vi "Set Channel Value and Get Buffer.vi"(8 "error in":errorcluster, 9 "Value":dbl, 10 "Channel":string, 11 "BufferWritesDBL in":refnum<class "BufferWrites1SamDBL.lvclass">) -> (0 "error out":errorcluster, 2 "Write Buffer":dbl[](array[numeric]), 3 "BufferWritesDBL out":refnum<class "BufferWrites1SamDBL.lvclass">)   [LabVIEW 2023, in "BufferWrites1SamDBL.lvclass"]
uses:
  BufferWrites1SamDBL.lvclass
  BufferWrites1SamDBL.lvclass/BufferWrites1SamDBL.ctl
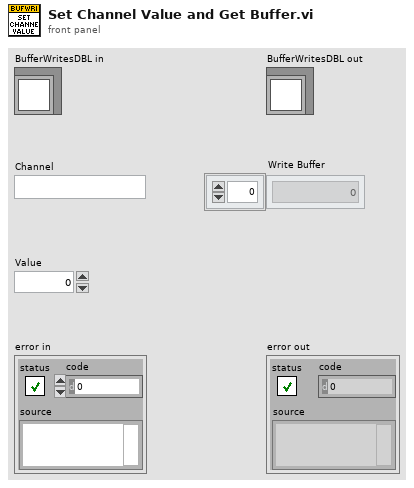
[diagram p1: front panel]
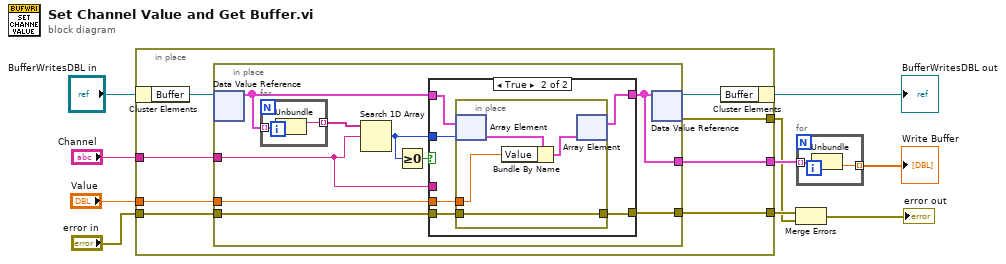
[diagram p0: block diagram]
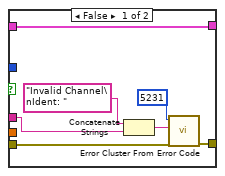
[diagram p2: hidden frame]
diagram:
  n1 = in-place {
    in-place-border: "Value" -> [w18]
    in-place-border: [w17] -> w1
    in-place-border: "Channel" -> [w16]
    in-place-border: [w13] -> w5
    in-place-border: "error in" -> [w12]
    in-place-border: [w11] -> w2
    n2 = in-place-cluster #1("BufferWritesDBL in") -> ("Buffer"=w15:refnum<data-value>)
    n3 = in-place {
      in-place-border: w18 -> [w27]
      in-place-border: w16 -> [w19]
      in-place-border: [w22] -> w13
      in-place-border: w12 -> [w21]
      in-place-border: [w20] -> w11
      n4 = in-place-dvr #2(w15) -> (w25:cluster{"Ident":string, "Value":dbl}[])  [unwired: 1 out]
      n5 = for {
        tunnel: w25 -> [w46] mode=indexing
        tunnel: [w45] -> w26 mode=indexing
        n6 = Unbundle(w46) -> ("Ident"=w45:string)  [unwired: 1 out]
      }
      n7 = Search 1D Array(1D array=w26, element=w19) -> (index of element=w23:i32)  [unwired: 1 in]
      n8 = Greater Or Equal To 0?(x=w23) -> (x >= 0?=w24:bool)
      n9 = case shown="True" w24 {
        tunnel: w27 -> [_ w40]
        tunnel: [w34 w39] -> w22
        tunnel: w25 -> [w34 w38]
        tunnel: w23 -> [_ w37]
        tunnel: w21 -> [w33 w36]
        tunnel: [w32 w35] -> w20
        tunnel: w19 -> [w28 _]
        frame False {
          n10 = Concatenate Strings("Invalid Channel\nIdent: " ("string"), w28) -> (w30:string)
          n11 = call <vilib>:"Error Cluster From Error Code.vi"("error in (no error)"=w33, "error message (\"\")"=w30, "error code (0)"=5231) -> ("error out"=w32:errorcluster)  [unwired: 6 in]
        }
        frame True {
          n12 = in-place {
            in-place-border: w40 -> [w42]
            in-place-border: w36 -> [w41]
            in-place-border: [w41] -> w35
            n13 = in-place-array #3(w38, w37) -> (w44:cluster{"Ident":string, "Value":dbl})
            n14 = Bundle By Name(cluster=w44, "Value"=w42) -> (w43:cluster{"Ident":string, "Value":dbl})
            n15 = in-place-array #3(w43) -> (w39:cluster{"Ident":string, "Value":dbl}[])  [unwired: 1 out]
          }
        }
      }
      n16 = in-place-dvr #2(w22) -> (w14:refnum<data-value>, w17:errorcluster)
    }
    n17 = in-place-cluster #1("Buffer"=w14) -> (→"BufferWritesDBL out":refnum<class "BufferWrites1SamDBL.lvclass">)
  }
  n18 = Merge Errors(w2, w1) -> (→"error out":errorcluster)
  n19 = for {
    tunnel: w5 -> [w48] mode=indexing
    tunnel: [w47] -> w4 mode=indexing
    n20 = Unbundle(w48) -> ("Value"=w47:dbl)  [unwired: 1 out]
  }
  "Write Buffer" <- w4
